vi "myRIO_BRig_RT_dataExp_ENL_max.vi"() -> (2 "output_ENL_max":i32)   [LabVIEW 2014]
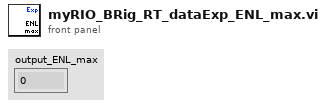
[diagram p1: front panel]
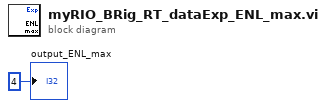
[diagram p0: block diagram]
diagram:
  "output_ENL_max" <- 4 ("output_iBlock")
